vi "Zadanie 3 odczyt z pliku.vi"() -> ()   [LabVIEW 2020]
uses:
  <vilib>/Utility/file.llb/Read Delimited Spreadsheet (DBL).vi
panel:
  out "XY Graph":cluster{"all rows":dbl[], "all rows":dbl[]}[](graph)
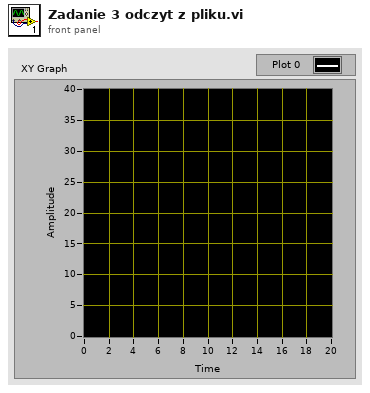
[diagram p1: front panel]
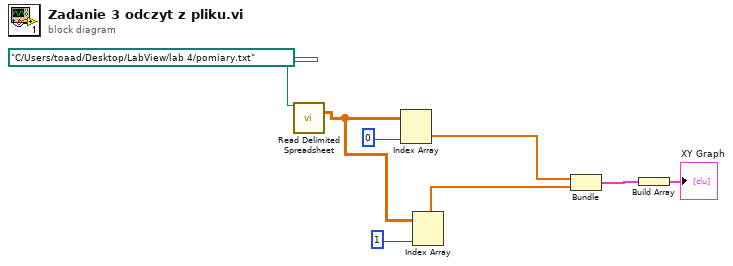
[diagram p0: block diagram]
diagram:
  n1 = call-poly <vilib>:"Read Delimited Spreadsheet.vi"("file path (dialog if empty)"=path "C:/Users/toaad/Desktop/LabView/lab 4/pomiary.txt" ("file (use dialog)")) -> ("all rows"=w5:dbl[][])  [unwired: 9 in, 5 out]
  n2 = Index Array(array=w5, index (col)=0 ("index (row)")) -> (element=w8:dbl[])  [unwired: 1 in]
  n3 = Index Array(array=w5, index (col)=1 ("index (row)")) -> (element=w4:dbl[])  [unwired: 1 in]
  n4 = Bundle("all rows"=w8, "all rows"=w4) -> (w7:cluster{"all rows":dbl[], "all rows":dbl[]})  [unwired: 1 in]
  n5 = Build Array(w7) -> (→"XY Graph":cluster{"all rows":dbl[], "all rows":dbl[]}[])
